vi "Initialize FPGA Resource.vi"(8 "Error In":errorcluster, 10 "FPGA VI Reference":T1, 11 "Display In":refnum<class "Display Manager.lvclass">) -> (0 "Error Out":errorcluster, 3 "Display Out":refnum<class "Display Manager.lvclass">)   [LabVIEW 2021]
uses:
  Display Manager.lvclass
  Controls/FPGA Reference.ctl
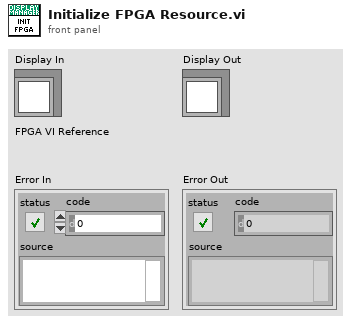
[diagram p1: front panel]
types:
  T1 = typedef "FPGA Reference.ctl" = refnum<k20>
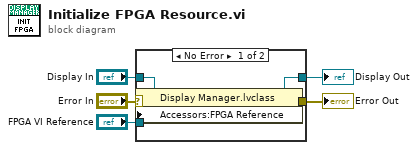
[diagram p0: block diagram]
diagram:
  n1 = case shown="No Error" "Error In" {
    selector: "Error In" -> [w10 w11]
    tunnel: "Display In" -> [w9 w12]
    tunnel: [w8 w12] -> w3
    tunnel: [w7 w11] -> w2
    tunnel: "FPGA VI Reference" -> [w6 _]
    frame No Error {
      n2 = property class="Display Manager.lvclass"(reference=w9, error in=w10, "Accessors:FPGA Reference"=w6) -> (reference out=w8:refnum<class "Display Manager.lvclass">, error out=w7:errorcluster)
    }
    frame Error {
    }
  }
  "Display Out" <- w3
  "Error Out" <- w2
